vi "LSX Get Slide.vi"(7 "mode":i32, 8 "error in (no error)":errorcluster, 9 "slot":i32, 10 "maga":i32, 11 "lLSID":i32) -> (0 "error out":errorcluster, 3 "function return":i32)   [LabVIEW 2016, in "Tango_DLL.lvlib"]
doc: "TANGOAPI int TANGOCALL LSX_GetSlide (int lLSID, int maga, int slot, int mode);"
uses:
  Tango_DLL.lvlib
  2017/Microscope Control/Device Library/Stages/Marzhauser/SCAN IM 120 x 80/Tango DLL VIs/Tango_DLL.dll
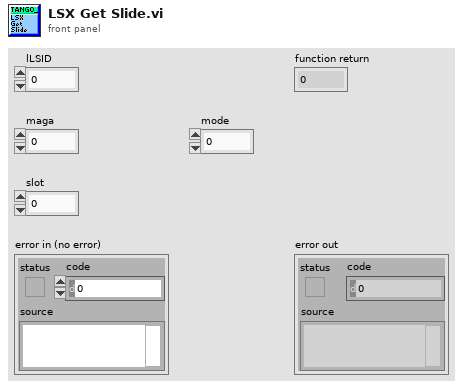
[diagram p1: front panel]
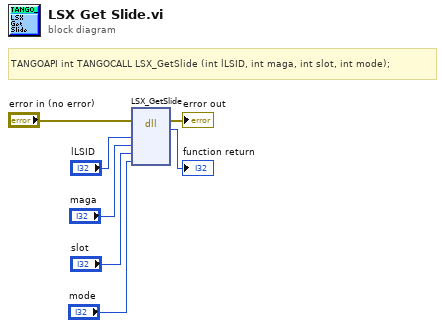
[diagram p0: block diagram]
diagram:
  # "TANGOAPI int TANGOCALL LSX_GetSlide (int lLSID, int maga, int slot, int mode);"
  n1 = dll-call lib="C:/Users/4PiSMS/Documents/Microscope Control/2017/Microscope Control/Device Library/Stages/Marzhauser/SCAN IM 120 x 80/Tango DLL VIs/Tango_DLL.*" fn="LSX_GetSlide"(error in="error in (no error)", "lLSID"="lLSID", "maga"="maga", "slot"="slot", "mode"="mode") -> (error out=→"error out":errorcluster, →"function return":i32)  [unwired: 6 in, 1 out]
